vi "Dbl Click Callback.vi"(4 "Net Data Event Ref":T1, 5 "Event Data":cluster{"dblClickedItem":T2}, 6 "Control Ref":T3, 7 "Event Common Data":T4) -> ()   [LabVIEW 2020, in "NI_VS UI Tree Alias Browser.lvlib"]
uses:
  <vilib>/NI VeriStand/UI Controls/Tree and Alias Browser/NI_VS UI Tree Alias Browser.lvlib
  <vilib>/NI VeriStand/UI Controls/Tree and Alias Browser/Tree Alias Browser Ref.ctl
  NationalInstruments.VeriStand.SystemStorageUI
  <vilib>/NI VeriStand/UI Controls/Tree and Alias Browser/Node Ref.ctl
  NationalInstruments.VeriStand.SystemStorage
  <vilib>/NI VeriStand/UI Controls/Tree and Alias Browser/Net Event Data Ref.ctl
  <vilib>/NI VeriStand/UI Controls/Tree and Alias Browser/Net Event Data.ctl
  <vilib>/NI VeriStand/UI Controls/Tree and Alias Browser/Net Event.ctl
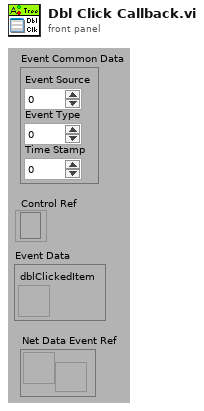
[diagram p1: front panel]
types:
  T1 = typedef "NI_VS UI Tree Alias Browser.lvlib/Net Event Data Ref.ctl" = refnum<user-event>
  T2 = typedef "NI_VS UI Tree Alias Browser.lvlib/Node Ref.ctl" = refnum<k24>
  T3 = typedef "NI_VS UI Tree Alias Browser.lvlib/Tree Alias Browser Ref.ctl" = refnum<k24>
  T4 = cluster{"Event Source":i32, "Event Type":u32, "Time Stamp":u32}
  T5 = typedef "NI_VS UI Tree Alias Browser.lvlib/Net Event Data.ctl" = cluster{"Type":T6, "Data":variant}
  T6 = typedef "NI_VS UI Tree Alias Browser.lvlib/Net Event.ctl" = enum16{"SelectedItem", "DblClick"}
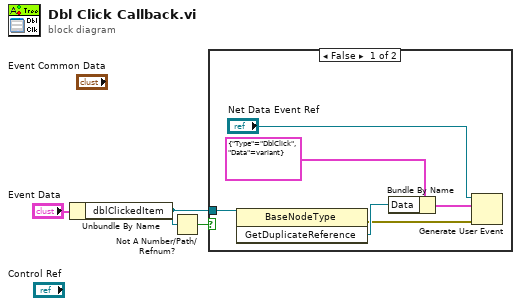
[diagram p0: block diagram]
diagram:
  n1 = Unbundle By Name("Event Data") -> ("dblClickedItem"=w2:T2)
  n2 = Not A Number/Path/Refnum?(number/path/refnum=w2) -> (NaN/Path/Refnum?=w1:bool)
  n3 = case shown="False" w1 {
    tunnel: w2 -> [w7 _]
    frame False {
      n4 = invoke class="BaseNodeType" method="GetDuplicateReference"(reference=w7) -> (error out=w5:errorcluster, "GetDuplicateReference"=w6:refnum<k24>)  [unwired: 2 in, 1 out]
      n5 = Bundle By Name(cluster=T5 {"Type"=enum."DblClick", "Data"=variant} ("event data"), "Data"=w6) -> (w8:T5)
      n6 = Generate User Event(user event="Net Data Event Ref", event data cluster=w8, error in=w5) -> ()  [unwired: 1 in, 2 out]
    }
    frame True {
    }
  }
